vi "Drive Immediate.vi"(0 "Left Setpoint":dbl, 2 "Description":string, 5 "Right Setpoint":dbl, 7 "Operation":T1, 9 "Deadband Value":dbl=0.01, 11 "Command Info In":T2, 12 "Transmition Engaged?":bool) -> (15 "Command Info Out":T2)   [LabVIEW 2019]
doc: "Often used for joystick control, this VI checks to see that the joystick axes are outside the deadband and updates the motors appropriately."
uses:
  <vilib>/Rock Robotics/WPI/Framework/Command Status Info.ctl
  <vilib>/Rock Robotics/WPI/Framework/Completion Status.ctl
  <vilib>/Rock Robotics/WPI/Framework/Completion Notifier.ctl
  Implementation/Drive Operations.ctl
  Implementation/Drive Setpoints.ctl
  Bordeaux/Command Stuff/Single Cmd Info.ctl
  <vilib>/picture/picture.llb/imagedata.ctl
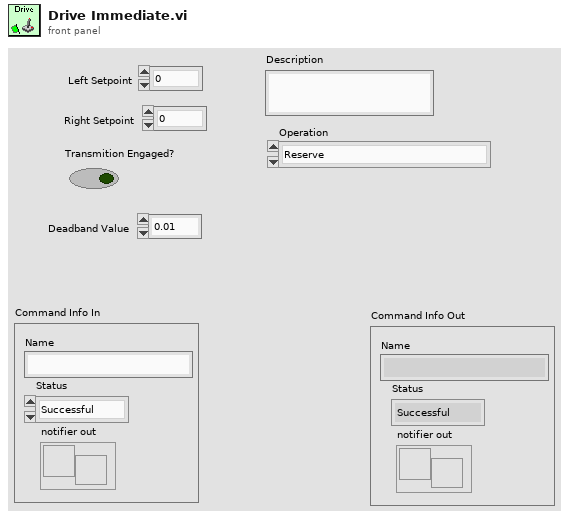
[diagram p1: front panel]
types:
  T1 = typedef "Drive Operations.ctl" = enum16{"Reserve", "Read Current", "Immediate", "Pod Racer", "Ball AA", "Play Back From Log"}
  T2 = typedef "Command Status Info.ctl" = cluster{"Name":string, "Status":T3, "notifier out":T4}
  T3 = typedef "Completion Status.ctl" = enum16{"Successful", "Aborted", "Incomplete"}
  T4 = typedef "Completion Notifier.ctl" = refnum<notifier>
  T5 = typedef "Drive Setpoints.ctl" = cluster{"Operation":T1, "Forwards/Backwards":dbl, "Turning":dbl, "Transmition Engaged?":bool, "Reverse (T) / Normal (F)":bool, "Field Align?":bool, "Auto Path Data":cluster{"V":dbl[], "Theta":dbl[], "Sample Period":dbl}, "Path Reversed":bool, "Commands":cluster{"Time (s)":dbl, T6, bool}[]}
  T6 = typedef "Single Cmd Info.ctl" = cluster{"Name":string, "CPTM.DataType":variant, "All Control Values Variant":cluster{"Name":string, "Variant Data":variant}[], "icon full":T7, "icon scaled":T7, "Path":path, "Subsystem Color":u32}
  T7 = typedef "imagedata.ctl" = cluster{"image type":i32, "image depth":i32, "image":u8[], "mask":u8[], "colors":u32[], "Rectangle":cluster{"left":i16, "top":i16, "right":i16, "bottom":i16}}
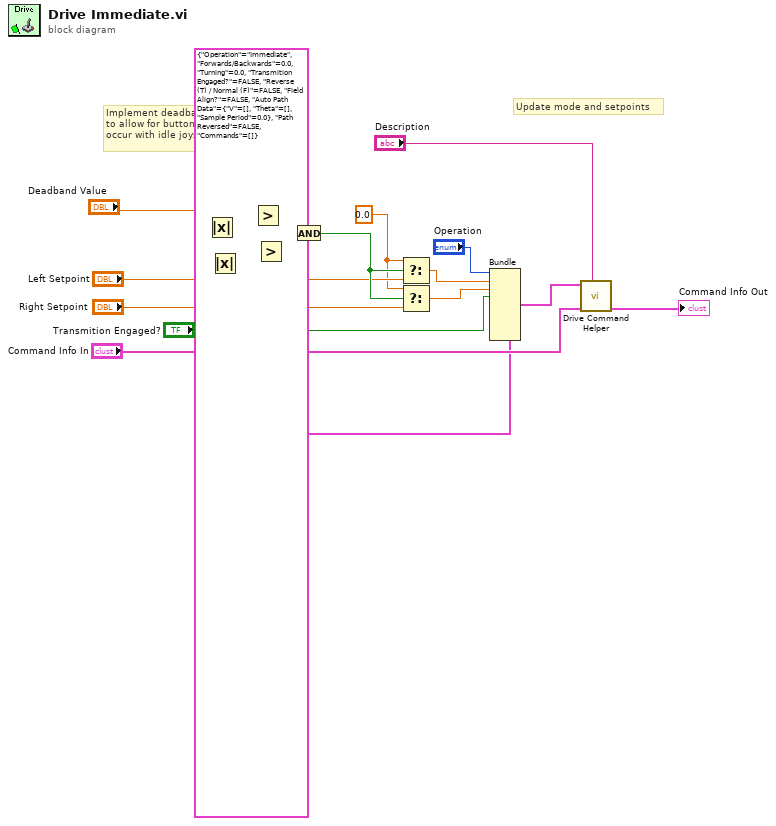
[diagram p0: block diagram]
diagram:
  w4 = 0.0 ("t")
  # "Implement deadband, mostly\nto allow for button driven operations\noccur with idle joysticks"
  # "Update mode and setpoints"
  n1 = Absolute Value(x="Left Setpoint") -> (abs(x)=w18:dbl)
  n2 = Absolute Value(x="Right Setpoint") -> (abs(x)=w12:dbl)
  n3 = Greater?(x="Deadband Value", y=w18) -> (0:w13:bool)
  n4 = Greater?(x="Deadband Value", y=w12) -> (0:w11:bool)
  n5 = And(x=w13, y=w11) -> (x .and. y?=w7:bool)
  n6 = Select(t=w4, s=w7, f="Left Setpoint") -> (s? t:f=w3:dbl)
  n7 = Select(t=w4, s=w7, f="Right Setpoint") -> (s? t:f=w2:dbl)
  n8 = Bundle(cluster=T5 {"Operation"=enum."Immediate", "Forwards/Backwards"=0.0, "Turning"=0.0, "Transmition Engaged?"=FALSE, "Reverse (T) / Normal (F)"=FALSE, "Field Align?"=FALSE, "Auto Path Data"={"V"=[], "Theta"=[], "Sample Period"=0.0}, "Path Reversed"=FALSE, "Commands"=[]} ("SubSystem Data"), "Operation"="Operation", "Forwards/Backwards"=w3, "Turning"=w2, "Transmition Engaged?"="Transmition Engaged?") -> (w8:T5)  [unwired: 5 in]
  n9 = call "Drive Command Helper.vi"("Description"="Description", "Command Info In"="Command Info In", "SubSystem Data"=w8) -> ("Command Info Out"=→"Command Info Out":T2)  [unwired: 6 in, 2 out]
